vi "AverageSampleHold.vi"(10 "Previous Average":i16, 11 "Input Value":i16) -> (2 "Output New Average":i16)   [LabVIEW 2015]
uses:
  <vilib>/rvi/Emulation/niFpgaEmulationIsFPGAContextNoSignature.vi
  <vilib>/rvi/Emulation/niFpgaSctlEmulationGetInTimedLoop.vi
  <vilib>/rvi/errors/niFpgaSetErrorForExecOnDevCompSimple.vi
  <vilib>/rvi/eio/common/nirviEmuReportErrorAndStop.vi
  <vilib>/rvi/DataTransferAndStorage/Container/Common/niFpgaContainerGetUniqueNameForEmu.vi
  <vilib>/rvi/FIFO/Fifo_Resource/nirvififoEmulationSetSize.vi
  <vilib>/rvi/FIFO/Fifo_Resource/nirviFifoEmulationQueueMgr.vi
  <instcachedir>/0/nirviFifoEmulationQueueMgr_E5CAEC123FF24DC58D834DCA3CDAA9B5.lvgen/nirviFifoEmulationQueueMgr_E5CAEC123FF24DC58D834DCA3CDAA9B5_001.vi
  <vilib>/Utility/error.llb/Clear Errors.vi
  <vilib>/rvi/FIFO/Fifo_Resource/nirvififoEmulationCreateLock.vi
  <vilib>/rvi/Emulation/niFpgaProcessEmulError.vi
  <vilib>/rvi/FIFO/Fifo_Resource/nirvififoEmulationObtainLock.vi
  <vilib>/rvi/FIFO/Fifo_Resource/nirvififoEmulationReleaseLock.vi
  <vilib>/rvi/occurrence/nirviWaitOnOccurrenceBase.vi
  <vilib>/rvi/errors/nirviReportUnexpectedCaseInternalError.vi
  <vilib>/rvi/errors/nirviReportUnexpectedCaseInternalError (U32).vi
  <vilib>/rvi/FIFO/Fifo_Resource/nirvififoEmulationDetermineInputValidOut.vi
  <vilib>/rvi/DataTransferAndStorage/Container/XNode/niFpgaContainer.xnode
  <vilib>/rvi/FIFO/Fifo_Resource/nirvififoEmulationRead.vi
  <vilib>/rvi/FIFO/Fifo_Resource/nirvififoEmulationWrite.vi
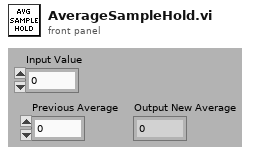
[diagram p1: front panel]
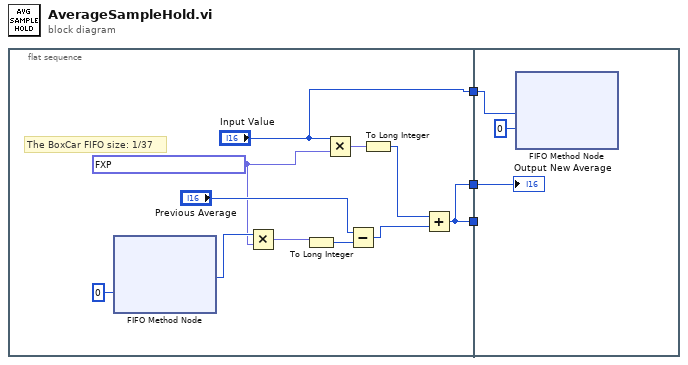
[diagram p0: block diagram]
diagram:
  n1 = flat-sequence {
    tunnel: ["Input Value"] -> w3
    tunnel: [w10] -> w2
    tunnel: [w10] -> w1
    tunnel: w3 -> [w17]
    tunnel: w2 -> [_]
    tunnel: w1 -> [w16]
    frame #0 {
      w7 = fxp<+,19,-5> 0.027027010917663574 ("y")
      # "The BoxCar FIFO size: 1/37"
      n2 = xnode ("FIFO Method Node")("Timeout"=0) -> ("Element"=w8:i32)  [unwired: 1 in, 2 out]
      n3 = Multiply(x=w8, y=w7) -> (x*y=w5:fxp<+/-,51,27>)
      n4 = To Long Integer(number=w5) -> (32bit integer=w6:i32)
      n5 = Multiply(x="Input Value", y=w7) -> (x*y=w12:fxp<+/-,35,11>)
      n6 = Subtract(x="Previous Average", y=w6) -> (x-y=w13:i32)
      n7 = To Long Integer(number=w12) -> (32bit integer=w11:i32)
      n8 = Add(x=w11, y=w13) -> (x+y=w10:i32)
    }
    frame #1 {
      n9 = xnode ("FIFO Method Node")("Element"=w17, "Timeout"=0) -> ()  [unwired: 1 in, 2 out]
      "Output New Average" <- w16
    }
  }
